vi "AboutGui.vi"() -> ()   [LabVIEW 2016]
uses:
  Global/ApplicationGlobal.vi
panel:
  out "Changelog":string="LASER MARKING\nT&M Solutions & Wabco\n----------------------------------------------------------------------------------------------\n" caption="MAKE CURRENT VALUE DEFAULT!!!"
  in  "OKButton":bool
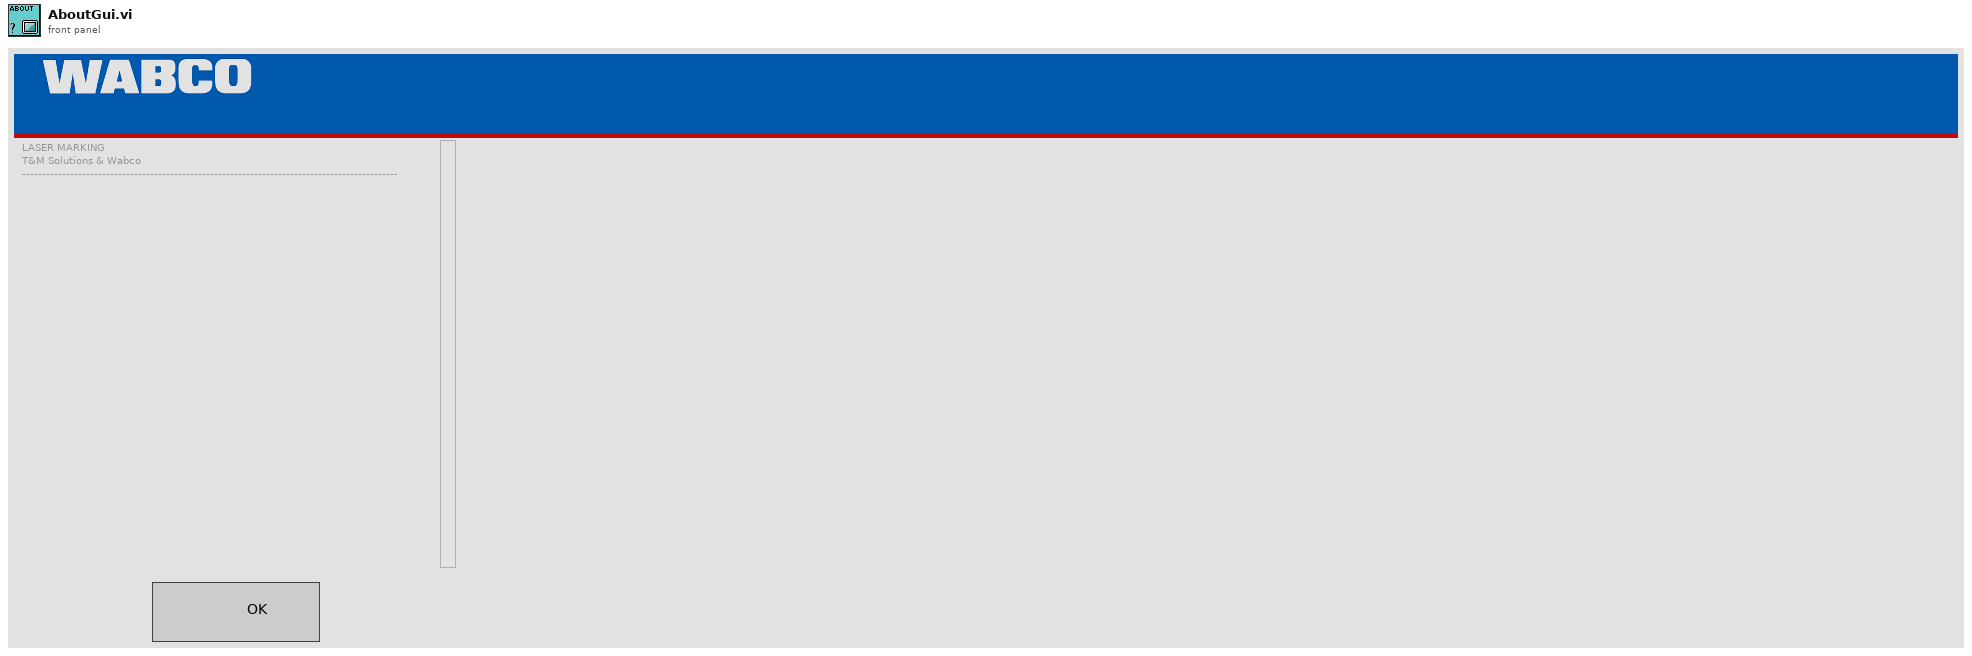
[diagram p1: front panel]
types:
  T1 = enum32{"Invalid", "Default", "Floating", "Floating/Auto-Hide", "Modal"}
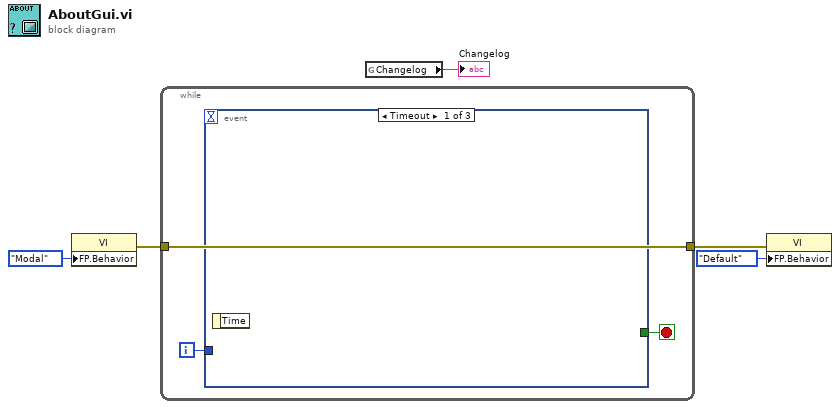
[diagram p0: block diagram]
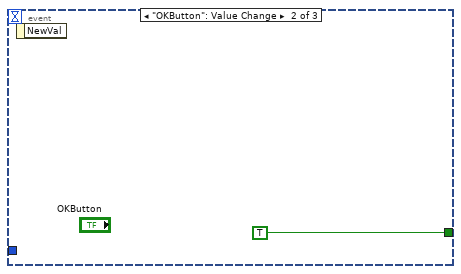
[diagram p2: hidden frame]
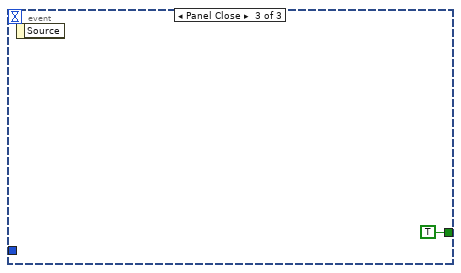
[diagram p3: hidden frame]
diagram:
  n1 = property class="VI"("FP.Behavior"=T1."Modal" ("Front Panel Window:Behavior")) -> (error out=w2:errorcluster)  [unwired: 2 in, 1 out]
  n2 = while "Respond to User" {
    tunnel: w2 -> [w6]
    tunnel: [w6] -> w1
    i -> [w7]
    stop <- w8 stop-if-true
    n3 = event shown="[0] Timeout" {
      selector: _ -> [_ _ _]
      dyn-events: _ -> [_ _ _]
      timeout: _ -> [_ _ _]
      tunnel: [_ TRUE TRUE] -> w8
      tunnel: w7 -> [_ _ _]
      event Timeout {
        n4 = event-data() -> ()  [unwired: 2 out]
      }
      event "OKButton": Value Change {
        n5 = event-data() -> ()  [unwired: 2 out]
      }
      event Panel Close {
        n6 = event-data() -> ()  [unwired: 2 out]
      }
    }
  }
  n7 = global read "ApplicationGlobal.vi" "Changelog"() -> (→"Changelog":string)
  n8 = property class="VI"(error in=w1, "FP.Behavior"=T1."Default" ("Front Panel Window:Behavior")) -> ()  [unwired: 1 in, 2 out]
